vi "Main.vi"() -> ()   [LabVIEW 2013]
uses:
  <vilib>/vision/Image Controls.llb/IMAQ Image.ctl
panel:
  in  "Non-tip Destination":path=path "C:/Users/Andrew/Documents/Apatite to Zircon Code/Track Finding/Tip Images/Non-Tips/unprocessed"
  in  "Tip Destination":path=path "C:/Users/Andrew/Documents/Apatite to Zircon Code/Track Finding/Tip Images/Tips/unprocessed"
  in  "Non-tips":T1[](array[plugin-control])
  in  "Tips":T1[](array[plugin-control])
  out "Files to Process":i32
  out "File Index":i32
  in  "Skip":bool
  in  "Image Array":T1[](array[typedef])
  in  "Stop":bool
  in  "Filenames":path[](array[path])
  out "Currently Processing:":string
  in  "Process Directory":bool
  in  "Process AVI":bool
  in  "Reset":bool
  in  "Save Samples":bool
  out "Progress":u8(slide) scale=0.0..100.0
  in  "Frame":i32(slide)
  in  "Current Image":T1(plugin-control)
  out "error out":errorcluster
  in  "error in (no error)":errorcluster
  # "AVI Processing"
  # "Extracted Samples"
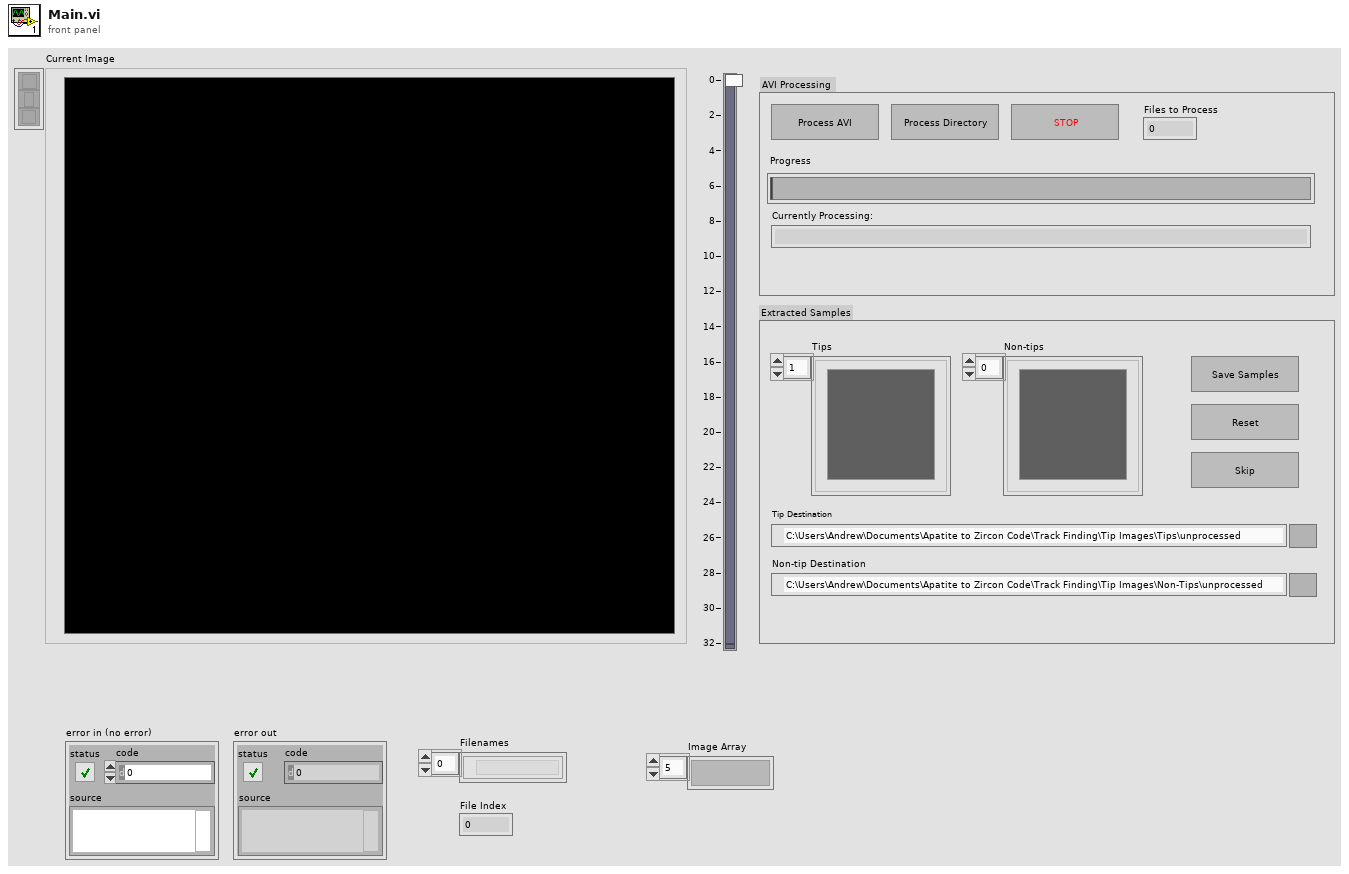
[diagram p1: front panel]
types:
  T1 = typedef "IMAQ Image.ctl" = refnum<image>
  T2 = enum8{"Enabled", "Disabled", "Disabled and Grayed Out"}
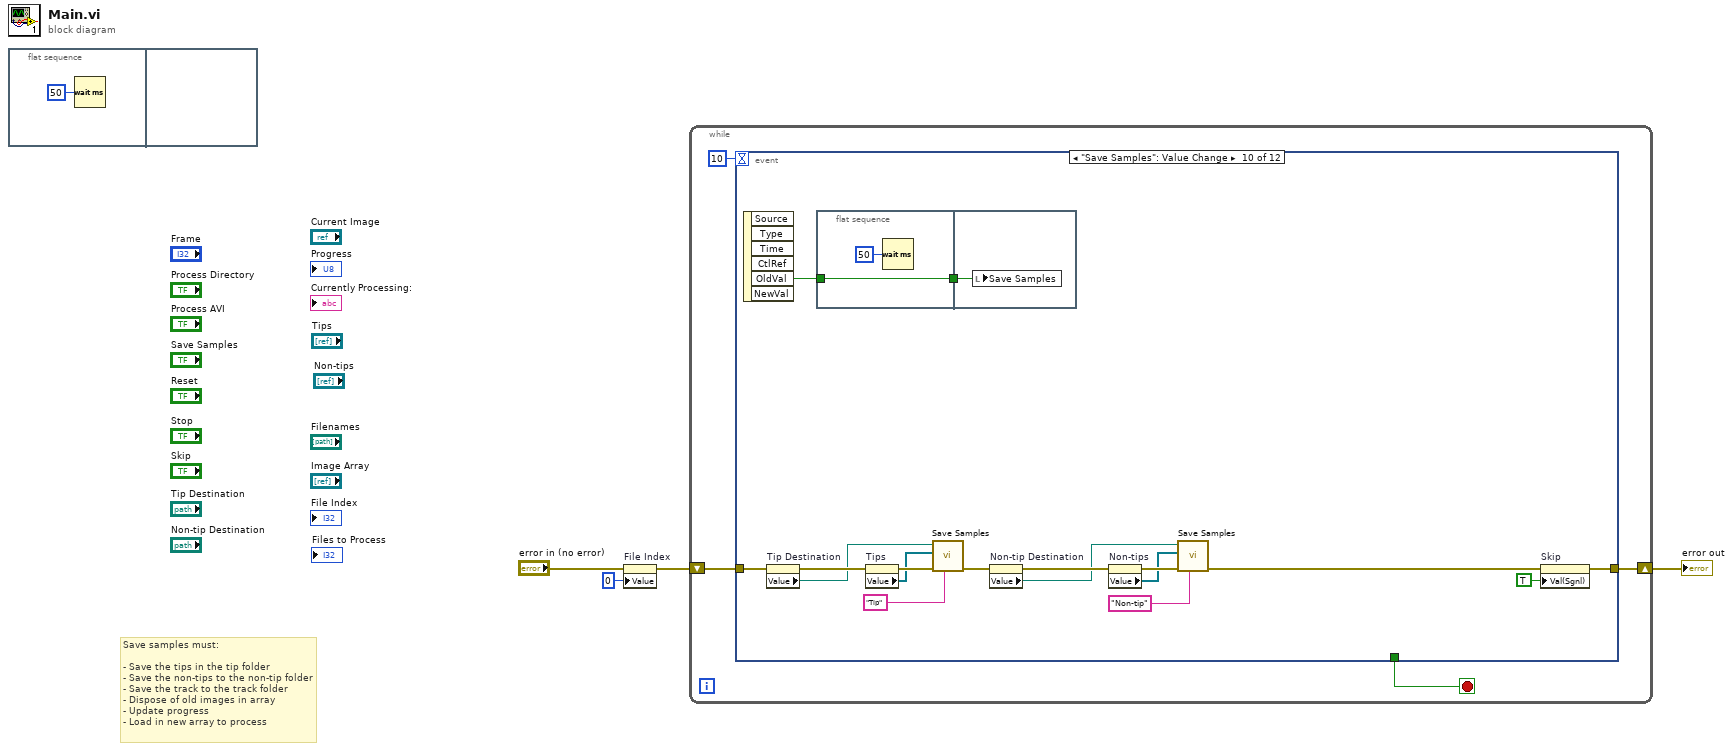
[diagram p0: block diagram]
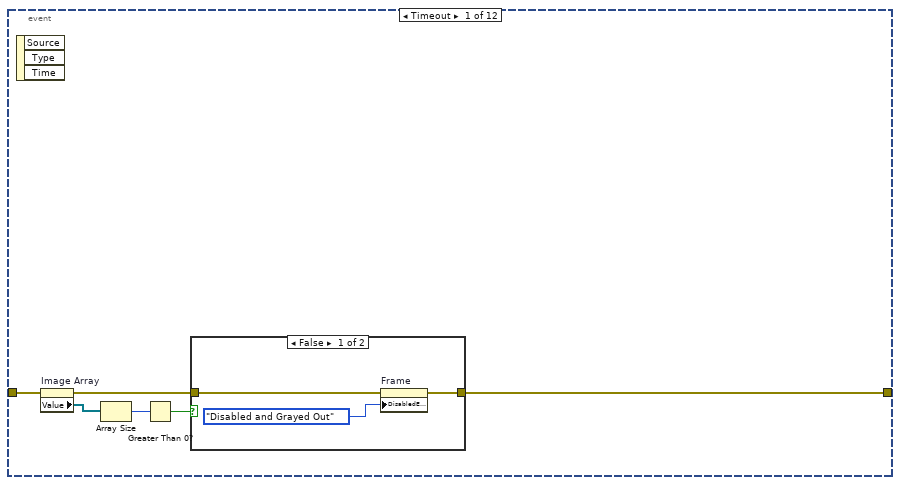
[diagram p2: hidden frame]
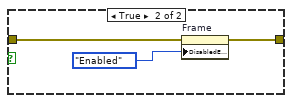
[diagram p3: hidden frame]
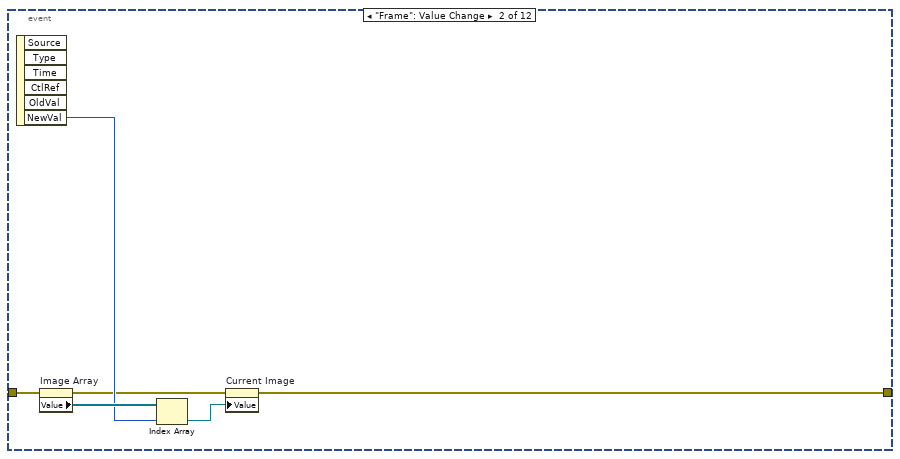
[diagram p4: hidden frame]
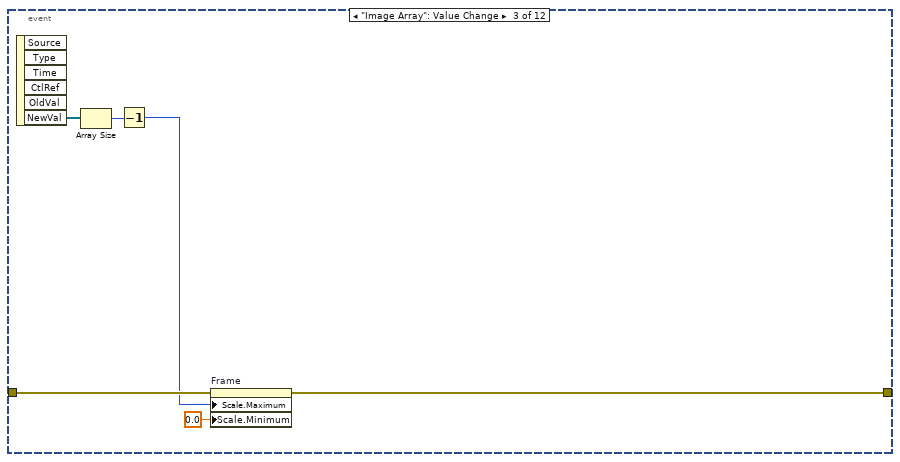
[diagram p5: hidden frame]
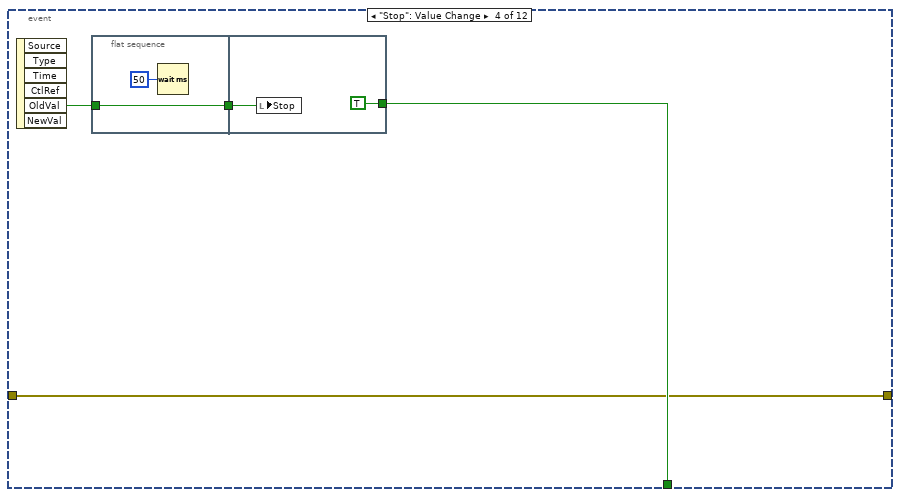
[diagram p6: hidden frame]
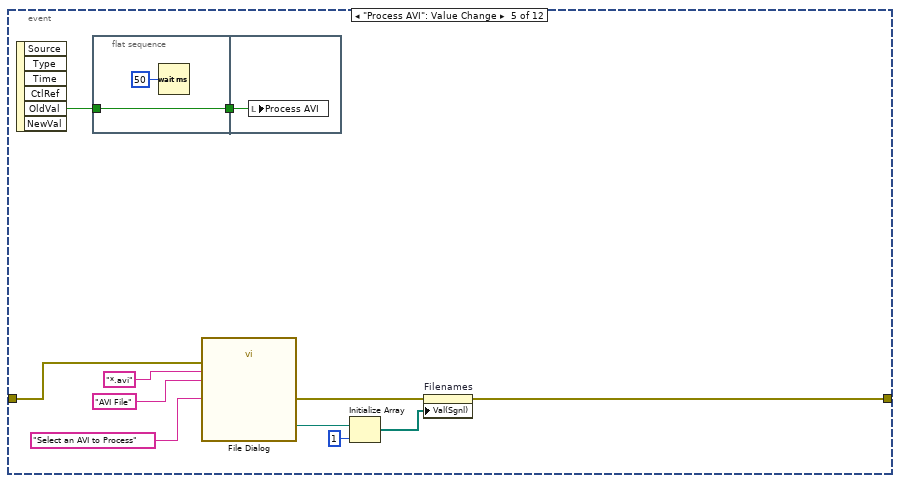
[diagram p7: hidden frame]
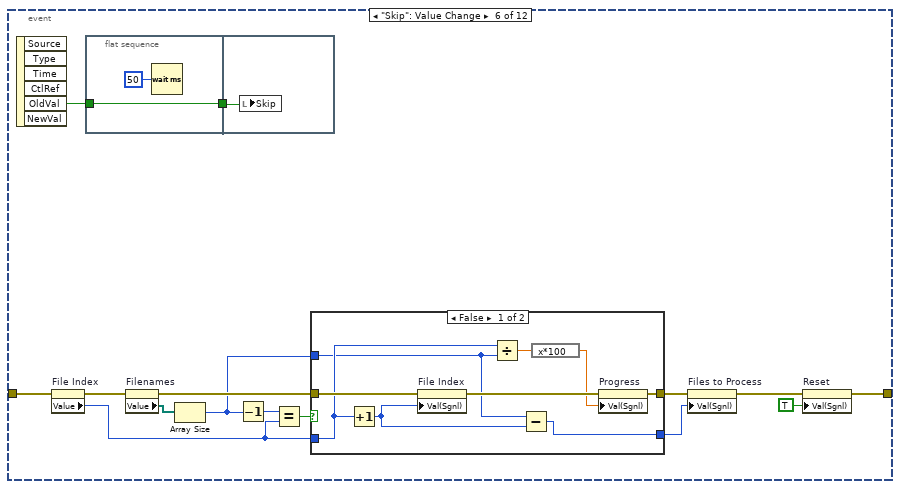
[diagram p8: hidden frame]
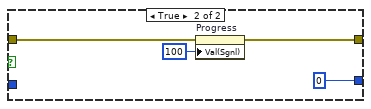
[diagram p9: hidden frame]
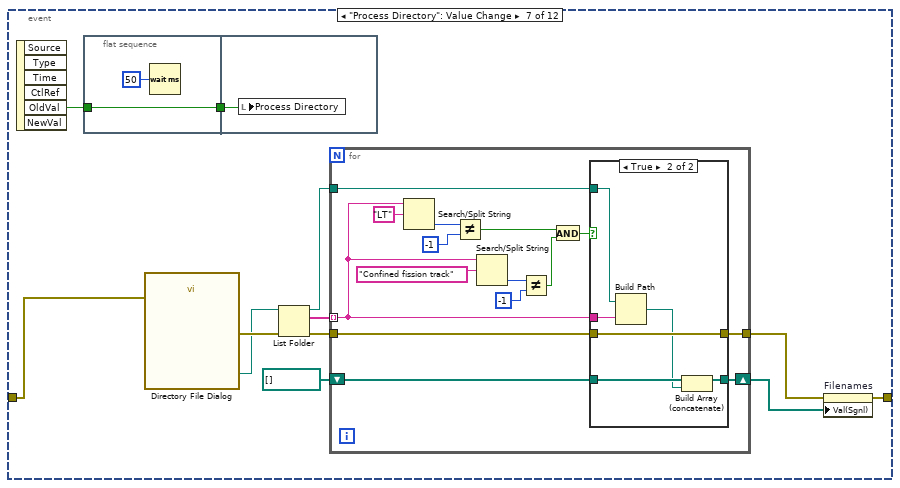
[diagram p10: hidden frame]
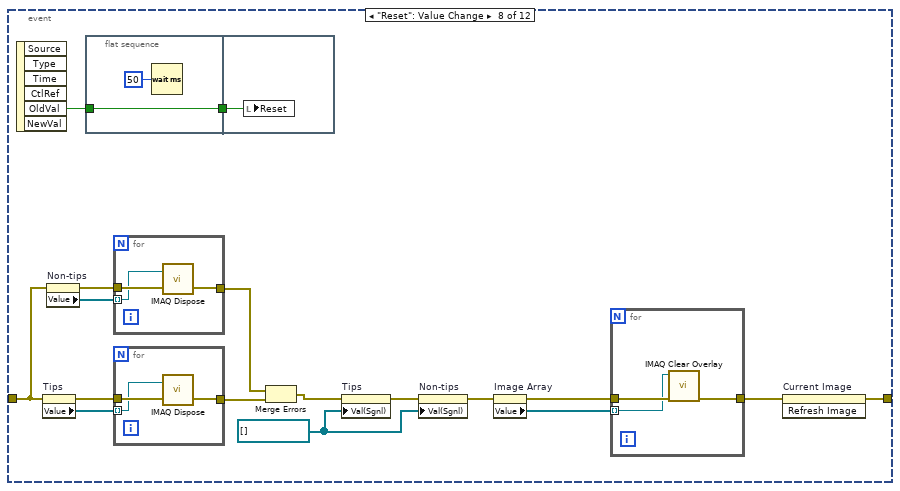
[diagram p12: hidden frame]
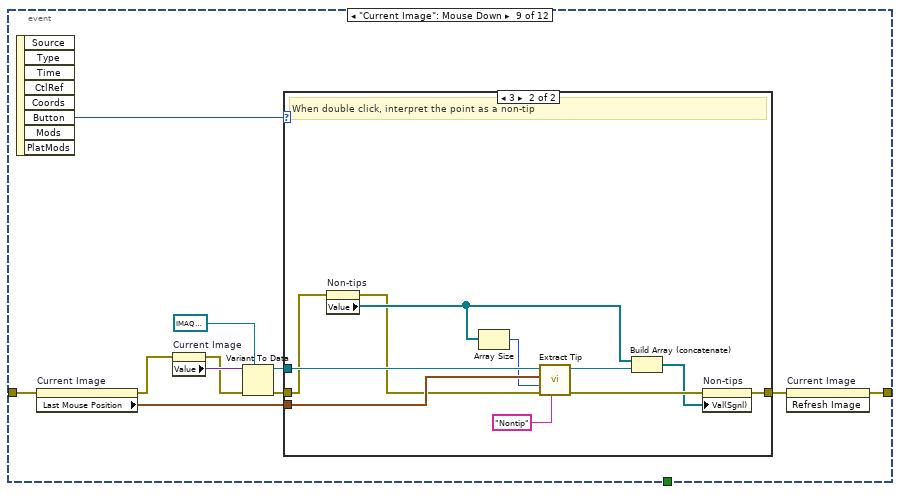
[diagram p13: hidden frame]
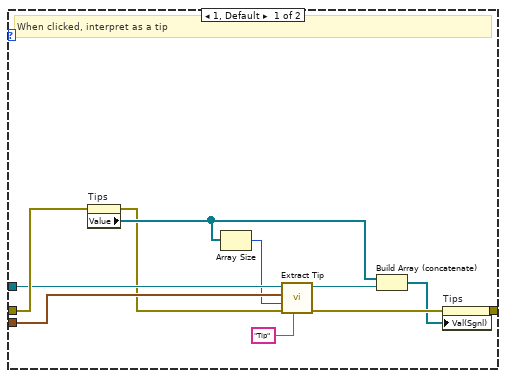
[diagram p14: hidden frame]
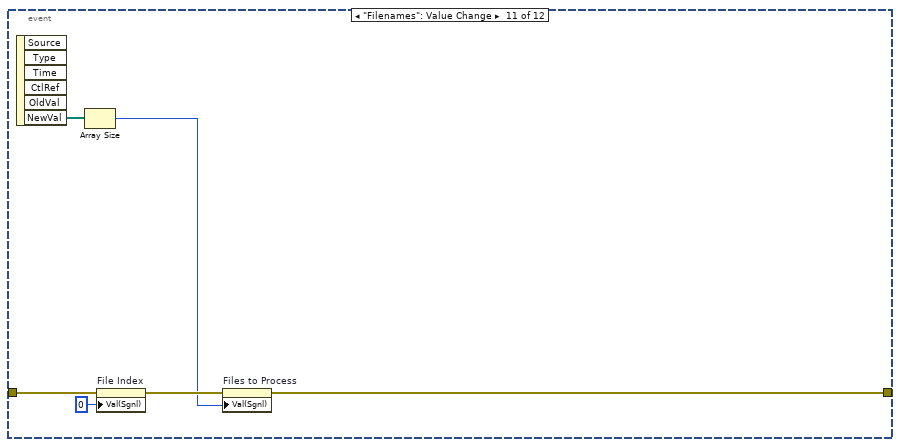
[diagram p15: hidden frame]
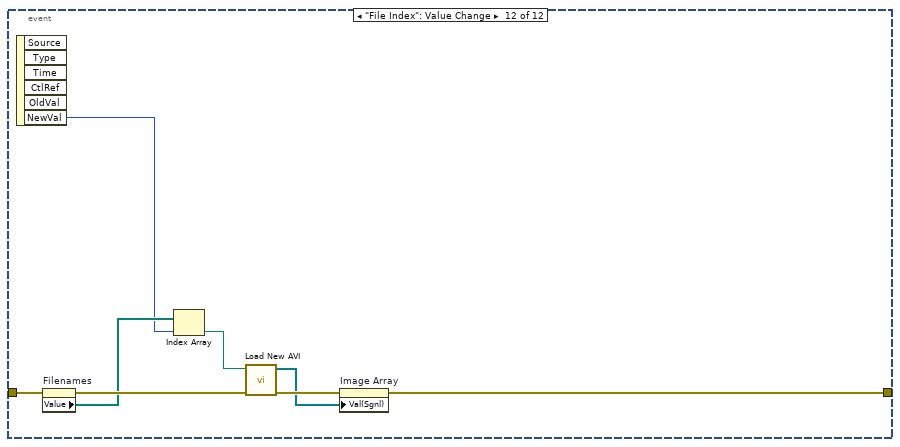
[diagram p16: hidden frame]
diagram:
  # "Save samples must:\n\n- Save the tips in the tip folder\n- Save the non-tips to the non-tip folder\n- Save the track to the track folder\n- Dispose of old images in array\n- Update progress\n- Load in new array to process"
  n1 = flat-sequence {
    frame #0 {
      n2 = Wait (ms)(milliseconds to wait=u32 50) -> ()  [unwired: 1 out]
    }
    frame #1 {
    }
  }
  n3 = property on="File Index" class="DigNum (strict)"(error in="error in (no error)", "Value"=0 ("File Index")) -> (error out=w3:errorcluster)  [unwired: 1 in, 1 out]
  n4 = while {
    shift-right: [w7] -> w4
    shift-left: w3 -> [w8]
    stop <- w9 stop-if-true
    n5 = event shown="[9] \"Save Samples\": Value Change" {
      selector: _ -> [_ _ _ _ _ _ _ _ _ _ _ _]
      dyn-events: _ -> [_ _ _ _ _ _ _ _ _ _ _ _]
      timeout: 10 -> [_ _ _ _ _ _ _ _ _ _ _ _]
      tunnel: [_ _ _ w35 _ _ _ _ _ _ _ _] -> w9
      tunnel: w8 -> [w15 w27 w33 w34 w50 w68 w96 w128 w164 w199 w212 w220]
      tunnel: [w10 w22 w29 w34 w43 w57 w91 w133 w154 w201 w207 w213] -> w7
      event Timeout {
        n6 = event-data() -> ()  [unwired: 1 in, 3 out]
        n7 = property on="Image Array" class="Arr (strict)"(error in=w15) -> (error out=w11:errorcluster, "Value"=w14:T1[])  [unwired: 1 in, 1 out]
        n8 = Array Size(array=w14) -> (size(s)=w13:i32)
        n9 = Greater Than 0?(x=w13) -> (x > 0?=w12:bool)
        n10 = case shown="False" w12 {
          tunnel: w11 -> [w18 w20]
          tunnel: [w17 w19] -> w10
          frame False {
            n11 = property on="Frame" class="Slide (strict)"(error in=w18, "DisabledEnum"=T2."Disabled and Grayed Out" ("Disabled")) -> (error out=w17:errorcluster)  [unwired: 1 in, 1 out]
          }
          frame True {
            n12 = property on="Frame" class="Slide (strict)"(error in=w20, "DisabledEnum"=T2."Enabled" ("Disabled")) -> (error out=w19:errorcluster)  [unwired: 1 in, 1 out]
          }
        }
      }
      event "Frame": Value Change {
        n13 = event-data() -> ("NewVal"=w25:i32)  [unwired: 1 in, 5 out]
        n14 = property on="Image Array" class="Arr (strict)"(error in=w27) -> (error out=w24:errorcluster, "Value"=w26:T1[])  [unwired: 1 in, 1 out]
        n15 = Index Array(array=w26, index=w25) -> (element=w23:T1)
        n16 = property on="Current Image" class="ImageControl"(error in=w24, "Value"=w23) -> (error out=w22:errorcluster)  [unwired: 1 in, 1 out]
      }
      event "Image Array": Value Change {
        n17 = event-data() -> ("NewVal"=w32:T1[])  [unwired: 1 in, 5 out]
        n18 = Array Size(array=w32) -> (size(s)=w31:i32)
        n19 = Decrement(x=w31) -> (x-1=w30:i32)
        n20 = property on="Frame" class="Slide (strict)"(error in=w33, "Scale.Maximum"=w30, "Scale.Minimum"=0.0 ("Scale.Range:Minimum")) -> (error out=w29:errorcluster)  [unwired: 1 in, 1 out]
      }
      event "Stop": Value Change {
        n21 = event-data() -> ("OldVal"=w37:bool)  [unwired: 1 in, 5 out]
        n22 = flat-sequence {
          tunnel: w37 -> [w38]
          tunnel: [w38] -> w36
          tunnel: w36 -> [w41]
          tunnel: [TRUE] -> w35
          frame #0 {
            n23 = Wait (ms)(milliseconds to wait=u32 50) -> ()  [unwired: 1 out]
          }
          frame #1 {
            n24 = local write "Stop"(w41) -> ()
          }
        }
      }
      event "Process AVI": Value Change {
        n25 = event-data() -> ("OldVal"=w52:bool)  [unwired: 1 in, 5 out]
        n26 = flat-sequence {
          tunnel: w52 -> [w53]
          tunnel: [w53] -> w51
          tunnel: w51 -> [w55]
          frame #0 {
            n27 = Wait (ms)(milliseconds to wait=u32 50) -> ()  [unwired: 1 out]
          }
          frame #1 {
            n28 = local write "Process AVI"(w55) -> ()
          }
        }
        n29 = call "File Dialog"("prompt"="Select an AVI to Process", "error in"=w50, "pattern (all files)"="*.avi", "pattern label"="AVI File") -> ("selected path"=w47:path, "error out"=w44:errorcluster)  [unwired: 8 in, 2 out]
        n30 = Initialize Array(w47, 1 ("dimension size")) -> (w45:path[])
        n31 = property on="Filenames" class="Arr (strict)"(error in=w44, "Val(Sgnl)"=w45) -> (error out=w43:errorcluster)  [unwired: 1 in, 1 out]
      }
      event "Skip": Value Change {
        n32 = event-data() -> ("OldVal"=w69:bool)  [unwired: 1 in, 5 out]
        n33 = property on="File Index" class="DigNum (strict)"(error in=w68) -> (error out=w67:errorcluster, "Value"=w63:i32)  [unwired: 1 in, 1 out]
        n34 = flat-sequence {
          tunnel: [w84] -> w70
          tunnel: w69 -> [w84]
          tunnel: w70 -> [w86]
          frame #0 {
            n35 = Wait (ms)(milliseconds to wait=u32 50) -> ()  [unwired: 1 out]
          }
          frame #1 {
            n36 = local write "Skip"(w86) -> ()
          }
        }
        n37 = property on="Filenames" class="Arr (strict)"(error in=w67) -> (error out=w65:errorcluster, "Value"=w66:path[])  [unwired: 1 in, 1 out]
        n38 = Array Size(array=w66) -> (size(s)=w61:i32)
        n39 = Decrement(x=w61) -> (x-1=w62:i32)
        n40 = Equal?(x=w62, y=w63) -> (x = y?=w64:bool)
        n41 = case shown="False" w64 {
          tunnel: w65 -> [w79 w83]
          tunnel: w63 -> [w73 _]
          tunnel: [w77 w82] -> w60
          tunnel: w61 -> [w71 _]
          tunnel: [w72 0] -> w59
          frame False {
            n42 = Increment(x=w73) -> (x+1=w74:i32)
            n43 = property on="File Index" class="DigNum (strict)"(error in=w79, "Val(Sgnl)"=w74) -> (error out=w78:errorcluster)  [unwired: 1 in, 1 out]
            n44 = Divide(x=w73, y=w71) -> (x/y=w76:dbl)
            n45 = Subtract(x=w71, y=w74) -> (x-y=w72:i32)
            n46 = expression code="x*100"(w76) -> (w75:dbl)
            n47 = property on="Progress" class="Slide (strict)"(error in=w78, "Val(Sgnl)"=w75) -> (error out=w77:errorcluster)  [unwired: 1 in, 1 out]
          }
          frame True {
            n48 = property on="Progress" class="Slide (strict)"(error in=w83, "Val(Sgnl)"=u8 100 ("Value (Signaling)")) -> (error out=w82:errorcluster)  [unwired: 1 in, 1 out]
          }
        }
        n49 = property on="Files to Process" class="DigNum (strict)"(error in=w60, "Val(Sgnl)"=w59) -> (error out=w58:errorcluster)  [unwired: 1 in, 1 out]
        n50 = property on="Reset" class="Bool (strict)"(error in=w58, "Val(Sgnl)"=TRUE ("Value (Signaling)")) -> (error out=w57:errorcluster)  [unwired: 1 in, 1 out]
      }
      event "Process Directory": Value Change {
        n51 = event-data() -> ("OldVal"=w98:bool)  [unwired: 1 in, 5 out]
        n52 = flat-sequence {
          tunnel: w98 -> [w122]
          tunnel: [w122] -> w97
          tunnel: w97 -> [w124]
          frame #0 {
            n53 = Wait (ms)(milliseconds to wait=u32 50) -> ()  [unwired: 1 out]
          }
          frame #1 {
            n54 = local write "Process Directory"(w124) -> ()
          }
        }
        n55 = call "Directory File Dialog"("error in"=w96) -> ("selected path"=w92:path, "error out"=w93:errorcluster)  [unwired: 11 in, 2 out]
        n56 = List Folder(path=w92, error in=w93) -> (path out=w90:path, filenames=w95:string[], error out=w94:errorcluster)  [unwired: 2 in, 1 out]
        n57 = for {
          tunnel: w95 -> [w102] mode=indexing
          tunnel: w94 -> [w108]
          shift-right: [w109] -> w88
          shift-left: path[] [] -> [w110]
          tunnel: [w107] -> w87
          tunnel: w90 -> [w106]
          n58 = Search/Split String(string=w102, search string/char (-)="LT") -> (offset of match=w113:i32)  [unwired: 1 in, 2 out]
          n59 = Not Equal?(x=w113, y=-1) -> (x != y?=w100:bool)
          n60 = Search/Split String(string=w102, search string/char (-)="Confined fission track") -> (offset of match=w103:i32)  [unwired: 1 in, 2 out]
          n61 = Not Equal?(x=w103, y=-1) -> (x != y?=w101:bool)
          n62 = And(x=w100, y=w101) -> (x .and. y?=w99:bool)
          n63 = case shown="True" w99 {
            tunnel: w110 -> [w114 w121]
            tunnel: [w114 w120] -> w109
            tunnel: w102 -> [_ w118]
            tunnel: w108 -> [w115 w119]
            tunnel: [w115 w119] -> w107
            tunnel: w106 -> [_ w117]
            frame False {
            }
            frame True {
              n64 = Build Path(base path=w117, name or relative path=w118) -> (appended path=w116:path)
              n65 = Build Array (concatenate)(w121, w116) -> (w120:path[])
            }
          }
        }
        n66 = property on="Filenames" class="Arr (strict)"(error in=w87, "Val(Sgnl)"=w88) -> (error out=w91:errorcluster)  [unwired: 1 in, 1 out]
      }
      event "Reset": Value Change {
        w138 = T1[] []
        n67 = event-data() -> ("OldVal"=w141:bool)  [unwired: 1 in, 5 out]
        n68 = property on="Tips" class="Arr (strict)"(error in=w128) -> (error out=w130:errorcluster, "Value"=w129:T1[])  [unwired: 1 in, 1 out]
        n69 = property on="Non-tips" class="Arr (strict)"(error in=w128) -> (error out=w132:errorcluster, "Value"=w131:T1[])  [unwired: 1 in, 1 out]
        n70 = flat-sequence {
          tunnel: w141 -> [w151]
          tunnel: [w151] -> w140
          tunnel: w140 -> [w153]
          frame #0 {
            n71 = Wait (ms)(milliseconds to wait=u32 50) -> ()  [unwired: 1 out]
          }
          frame #1 {
            n72 = local write "Reset"(w153) -> ()
          }
        }
        n73 = for {
          tunnel: w132 -> [w147]
          tunnel: w131 -> [w146] mode=indexing
          tunnel: [w145] -> w125
          n74 = call "IMAQ Dispose"("Image"=w146, "error in (no error)"=w147) -> ("error out"=w145:errorcluster)  [unwired: 4 in]
        }
        n75 = for {
          tunnel: w130 -> [w144]
          tunnel: w129 -> [w143] mode=indexing
          tunnel: [w142] -> w127
          n76 = call "IMAQ Dispose"("Image"=w143, "error in (no error)"=w144) -> ("error out"=w142:errorcluster)  [unwired: 4 in]
        }
        n77 = Merge Errors(w125, w127) -> (w126:errorcluster)
        n78 = property on="Tips" class="Arr (strict)"(error in=w126, "Val(Sgnl)"=w138) -> (error out=w139:errorcluster)  [unwired: 1 in, 1 out]
        n79 = property on="Non-tips" class="Arr (strict)"(error in=w139, "Val(Sgnl)"=w138) -> (error out=w137:errorcluster)  [unwired: 1 in, 1 out]
        n80 = property on="Image Array" class="Arr (strict)"(error in=w137) -> (error out=w135:errorcluster, "Value"=w136:T1[])  [unwired: 1 in, 1 out]
        n81 = for {
          tunnel: w136 -> [w149] mode=indexing
          tunnel: w135 -> [w150]
          tunnel: [w148] -> w134
          n82 = call "IMAQ Clear Overlay"("error in (no error)"=w150, "Image"=w149) -> ("error out"=w148:errorcluster)  [unwired: 8 in, 1 out]
        }
        n83 = invoke on="Current Image" class="ImageControl" method="Refresh Image"(error in=w134) -> (error out=w133:errorcluster)  [unwired: 2 in, 2 out]
      }
      event "Current Image": Mouse Down {
        n84 = event-data() -> ("Button"=w156:u16)  [unwired: 1 in, 7 out]
        n85 = property on="Current Image" class="ImageControl"(error in=w164) -> (error out=w162:errorcluster, "Last Mouse Position"=w163:cluster{"X":i32, "Y":i32})  [unwired: 1 in, 1 out]
        n86 = property on="Current Image" class="ImageControl"(error in=w162) -> (error out=w159:errorcluster, "Value"=w160:variant)  [unwired: 1 in, 1 out]
        n87 = Variant To Data(error in=w159, type=T1 refnum ("Tip 1"), Variant=w160) -> (data=w157:T1, error out=w161:errorcluster)
        n88 = case shown="3" w156 {
          tunnel: w161 -> [w173 w183]
          tunnel: w163 -> [w175 w186]
          tunnel: w157 -> [w172 w184]
          tunnel: [w170 w178] -> w155
          frame 1, Default {
            # "When clicked, interpret as a tip"
            n89 = property on="Tips" class="Arr (strict)"(error in=w173) -> (error out=w165:errorcluster, "Value"=w166:T1[])  [unwired: 1 in, 1 out]
            n90 = Array Size(array=w166) -> (size(s)=w171:i32)
            n91 = call "Extract Tip.vi"("Label"="Tip", "error in (no error)"=w165, "Tip Number"=w171, "Mouse Position"=w175, "Image"=w172) -> ("error out"=w169:errorcluster, "Tip Image"=w168:T1)  [unwired: 5 in]
            n92 = Build Array (concatenate)(w166, w168) -> (w167:T1[])
            n93 = property on="Tips" class="Arr (strict)"(error in=w169, "Val(Sgnl)"=w167) -> (error out=w170:errorcluster)  [unwired: 1 in, 1 out]
          }
          frame 3 {
            # "When double click, interpret the point as a non-tip"
            n94 = property on="Non-tips" class="Arr (strict)"(error in=w183) -> (error out=w176:errorcluster, "Value"=w177:T1[])  [unwired: 1 in, 1 out]
            n95 = Array Size(array=w177) -> (size(s)=w182:i32)
            n96 = call "Extract Tip.vi"("Label"="Nontip", "error in (no error)"=w176, "Tip Number"=w182, "Mouse Position"=w186, "Image"=w184) -> ("error out"=w181:errorcluster, "Tip Image"=w180:T1)  [unwired: 5 in]
            n97 = Build Array (concatenate)(w177, w180) -> (w179:T1[])
            n98 = property on="Non-tips" class="Arr (strict)"(error in=w181, "Val(Sgnl)"=w179) -> (error out=w178:errorcluster)  [unwired: 1 in, 1 out]
          }
        }
        n99 = invoke on="Current Image" class="ImageControl" method="Refresh Image"(error in=w155) -> (error out=w154:errorcluster)  [unwired: 2 in, 2 out]
      }
      event "Save Samples": Value Change {
        n100 = event-data() -> ("OldVal"=w203:bool)  [unwired: 1 in, 5 out]
        n101 = property on="Tip Destination" class="Path"(error in=w199) -> (error out=w198:errorcluster, "Value"=w197:path)  [unwired: 1 in, 1 out]
        n102 = flat-sequence {
          tunnel: w203 -> [w204]
          tunnel: [w204] -> w202
          tunnel: w202 -> [w206]
          frame #0 {
            n103 = Wait (ms)(milliseconds to wait=u32 50) -> ()  [unwired: 1 out]
          }
          frame #1 {
            n104 = local write "Save Samples"(w206) -> ()
          }
        }
        n105 = property on="Tips" class="Arr (strict)"(error in=w198) -> (error out=w196:errorcluster, "Value"=w195:T1[])  [unwired: 1 in, 1 out]
        n106 = call "Save Samples.vi"("Type of Feature"="Tip", "error in (no error)"=w196, "Images"=w195, "Destination Folder"=w197) -> ("error out"=w193:errorcluster)  [unwired: 7 in]
        n107 = property on="Non-tip Destination" class="Path"(error in=w193) -> (error out=w192:errorcluster, "Value"=w191:path)  [unwired: 1 in, 1 out]
        n108 = property on="Non-tips" class="Arr (strict)"(error in=w192) -> (error out=w190:errorcluster, "Value"=w189:T1[])  [unwired: 1 in, 1 out]
        n109 = call "Save Samples.vi"("Type of Feature"="Non-tip", "error in (no error)"=w190, "Images"=w189, "Destination Folder"=w191) -> ("error out"=w187:errorcluster)  [unwired: 7 in]
        n110 = property on="Skip" class="Bool (strict)"(error in=w187, "Val(Sgnl)"=TRUE ("Value (Signaling)")) -> (error out=w201:errorcluster)  [unwired: 1 in, 1 out]
      }
      event "Filenames": Value Change {
        n111 = event-data() -> ("NewVal"=w210:path[])  [unwired: 1 in, 5 out]
        n112 = Array Size(array=w210) -> (size(s)=w208:i32)
        n113 = property on="File Index" class="DigNum (strict)"(error in=w212, "Val(Sgnl)"=0 ("Value (Signaling)")) -> (error out=w209:errorcluster)  [unwired: 1 in, 1 out]
        n114 = property on="Files to Process" class="DigNum (strict)"(error in=w209, "Val(Sgnl)"=w208) -> (error out=w207:errorcluster)  [unwired: 1 in, 1 out]
      }
      event "File Index": Value Change {
        n115 = event-data() -> ("NewVal"=w214:i32)  [unwired: 1 in, 5 out]
        n116 = property on="Filenames" class="Arr (strict)"(error in=w220) -> (error out=w216:errorcluster, "Value"=w215:path[])  [unwired: 1 in, 1 out]
        n117 = Index Array(array=w215, index=w214) -> (element=w219:path)
        n118 = call "Load New AVI.vi"("error in (no error)"=w216, "AVI Path"=w219) -> ("error out"=w218:errorcluster, "Image Array"=w217:T1[])  [unwired: 8 in]
        n119 = property on="Image Array" class="Arr (strict)"(error in=w218, "Val(Sgnl)"=w217) -> (error out=w213:errorcluster)  [unwired: 1 in, 1 out]
      }
    }
  }
  "error out" <- w4
